vi "打开关闭通讯.vi"(8 "error in (no error)":errorcluster, 11 "功能输入":enum16{"打开串口", "关闭串口"}(ring)) -> (0 "error out":errorcluster, 3 "MB_Serial session":refnum<class "MB_Master_Serial.lvclass">)   [LabVIEW 2016, in "MGG-KL-QC流量计.lvlib"]
uses:
  <vilib>/Plasmionique/MB Master/MB_Master_Serial/MB_Master_Serial.lvclass
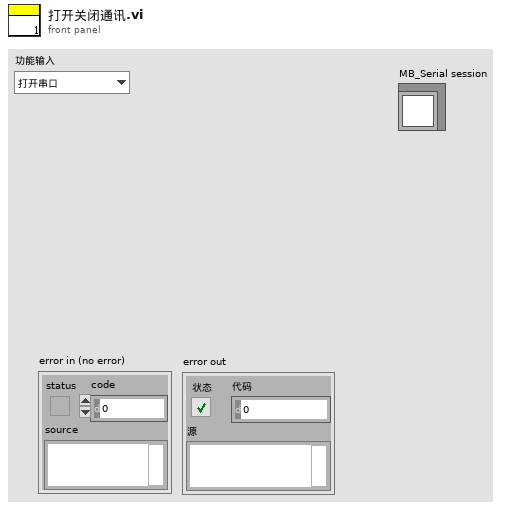
[diagram p1: front panel]
types:
  T1 = cluster{"baud rate (bps)":u32, "stop bits":u16, "parity":u16, "flow control":u16, "timeout":u32, "retries":i32}
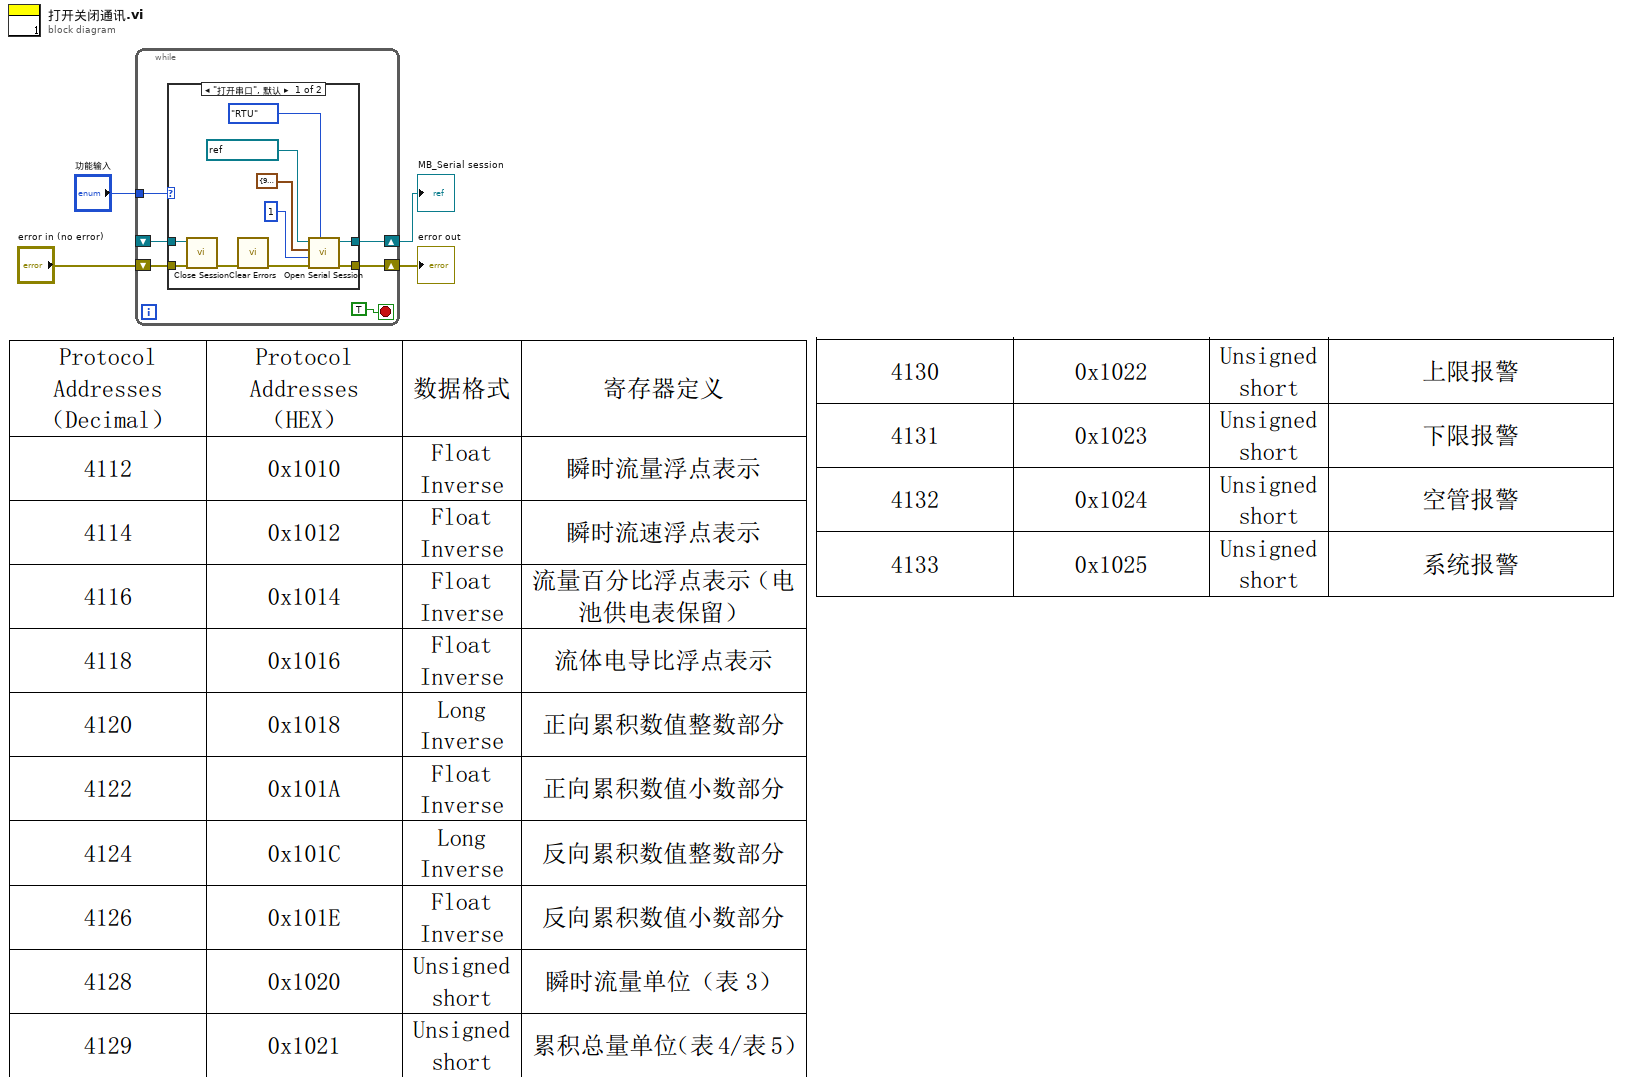
[diagram p0: block diagram]
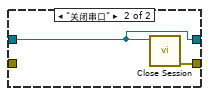
[diagram p2: hidden frame]
diagram:
  n1 = while {
    shift-right: [w9] -> w1
    shift-left: _ -> [w7]
    shift-right: [w8] -> w2
    shift-left: "error in (no error)" -> [w6]
    tunnel: "功能输入" -> [w5]
    stop <- TRUE stop-if-true
    n2 = case shown="\"打开串口\", 默认" w5 {
      tunnel: [w16 w21] -> w9
      tunnel: [w15 w22] -> w8
      tunnel: w7 -> [w14 w21]
      tunnel: w6 -> [w13 _]
      frame "打开串口", Default {
        n3 = call-dynamic "Close Session.vi"("error in (no error)"=w13, "MB_Serial session"=w14) -> ("error out"=w12:errorcluster)  [unwired: 9 in]
        n4 = call <vilib>:"Clear Errors.vi"("error in (no error)"=w12) -> ("error out"=w11:errorcluster)  [unwired: 5 in, 1 out]
        n5 = call <vilib>:"Open Serial Session.vi"("Mode (RTU)"=enum16{"RTU", "ASCII"}."RTU", "Error in"=w11, "Slave ID"=u8 1, "Serial Config"=T1 {"baud rate (bps)"=9600, "stop bits"=10, "parity"=0, "flow control"=0, "timeout"=1000, "retries"=1}, "VISA Resource"=refnum<visa-resource-name> "COM10") -> ("Error out"=w15:errorcluster, "MB_Serial session"=w16:refnum<class "MB_Master_Serial.lvclass">)  [unwired: 5 in]
      }
      frame "关闭串口" {
        n6 = call-dynamic "Close Session.vi"("MB_Serial session"=w21) -> ("error out"=w22:errorcluster)  [unwired: 10 in]
      }
    }
  }
  "error out" <- w2
  "MB_Serial session" <- w1
